vi "L1.1.vi"() -> ()   [LabVIEW 2020]
panel:
  out "Tono 6":dbl
  out "Tono 5":dbl
  out "Tono 4":dbl
  out "Tono 3":dbl
  out "Tono 2":dbl
  out "Tono 1":dbl
  out "DFT (N=64)":dbl[](graph)
  out "6":bool
  out "5":bool
  out "4":bool
  out "3":bool
  out "2":bool
  out "1":bool
  out "DFT (N=512)":dbl[](graph)
  in  "DFT  size":i32=-1
  in  "Canal DA myDAQ":tag="myDAQ1/audioOutputLeft"
  out "error out":errorcluster
  out "myDAQ lectura wav":dbl[](graph)
  in  "Canal AD myDAQ":tag="myDAQ1/audioInputLeft"
  in  "stop":bool
  in  "fs AD (Hz) myDAQ":dbl=50000.0 min=0.0 max=50000.0
  in  "numero de muestras myDAQ":i32
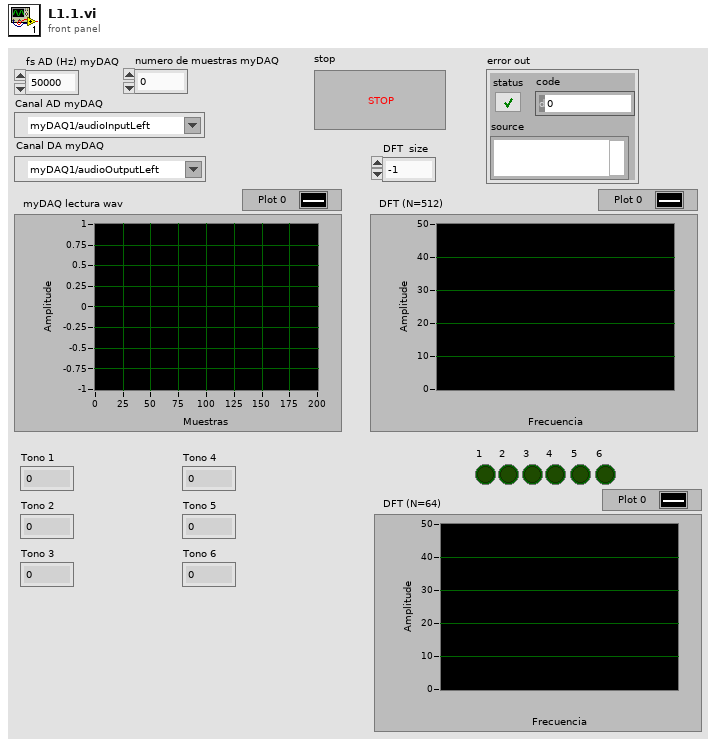
[diagram p1: front panel]
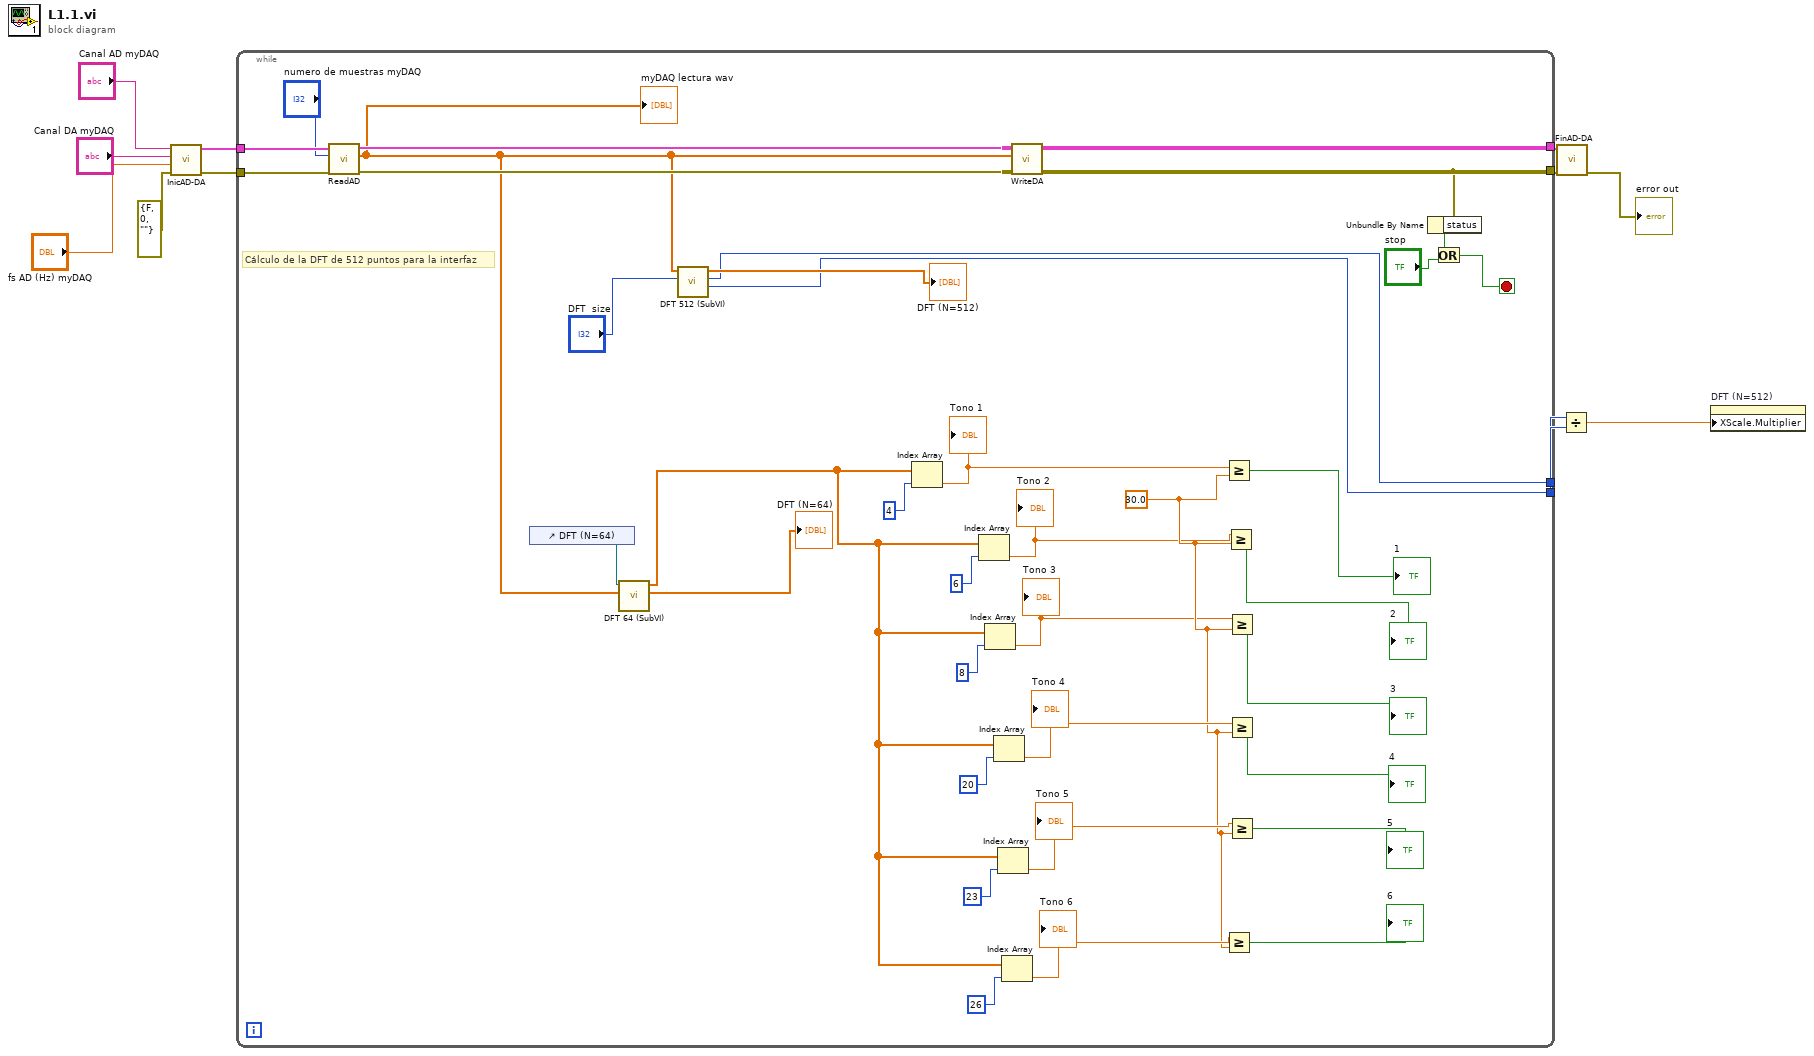
[diagram p0: block diagram]
diagram:
  n1 = call <userlib>:"InicAD-DA.vi"("error in"=errorcluster {"status"=FALSE, "code"=0, "source"=""}, "fs AD (Hz)"="fs AD (Hz) myDAQ", "Canal DA"="Canal DA myDAQ", "Canal AD"="Canal AD myDAQ") -> ("error out"=w9:errorcluster, "Tarea Out"=w10:cluster{"AD":refnum<k21>, "DA":refnum<k21>})  [unwired: 6 in]
  n2 = while {
    tunnel: [w41] -> w12
    tunnel: [w47] -> w11
    tunnel: w10 -> [w46]
    tunnel: w9 -> [w45]
    tunnel: [w38] -> w2
    tunnel: [w37] -> w1
    stop <- w43 stop-if-true
    w24 = 30.0 ("y")
    # "Cálculo de la DFT de 512 puntos para la interfaz"
    n3 = call <userlib>:"ReadAD.vi"("error in"=w45, "numero de muestras"="numero de muestras myDAQ", "Tarea In"=w46) -> ("error out"=w48:errorcluster, "Datos"=w36:dbl[], "Tarea Out"=w49:cluster{"AD":refnum<k21>, "DA":refnum<k21>})  [unwired: 6 in]
    "myDAQ lectura wav" <- w36
    n4 = control-ref of="DFT (N=64)"() -> (w14:refnum<vi>)
    n5 = call "DFT 64 (SubVI).vi"("Datos"=w36, "WaveformGraph in"=w14) -> ("DFT (N=64)"=→"DFT (N=64)":dbl[], "Array"=w29:dbl[])  [unwired: 8 in]
    n6 = call "DFT 512 (SubVI).vi"("DFT  size in"="DFT  size", "Datos"=w36) -> ("DFT  size out"=w38:i32, "x"=w37:i32, "Array"=→"DFT (N=512)":dbl[])  [unwired: 7 in]
    n7 = Index Array(array=w29, index=4) -> (element=w28:dbl)
    "Tono 1" <- w28
    n8 = Index Array(array=w29, index=6) -> (element=w17:dbl)
    "Tono 2" <- w17
    n9 = Index Array(array=w29, index=8) -> (element=w16:dbl)
    "Tono 3" <- w16
    n10 = Index Array(array=w29, index=20) -> (element=w25:dbl)
    "Tono 4" <- w25
    n11 = Index Array(array=w29, index=23) -> (element=w26:dbl)
    "Tono 5" <- w26
    n12 = Index Array(array=w29, index=26) -> (element=w27:dbl)
    "Tono 6" <- w27
    n13 = call <userlib>:"WriteDA.vi"("error in"=w48, "Datos"=w36, "Tarea In"=w49) -> ("error out"=w41:errorcluster, "Tarea Out"=w47:cluster{"AD":refnum<k21>, "DA":refnum<k21>})  [unwired: 7 in]
    n14 = Greater Or Equal?(x=w28, y=w24) -> (x >= y?=→"1":bool)
    n15 = Greater Or Equal?(x=w27, y=w24) -> (x >= y?=→"6":bool)
    n16 = Greater Or Equal?(x=w17, y=w24) -> (x >= y?=→"2":bool)
    n17 = Greater Or Equal?(x=w16, y=w24) -> (x >= y?=→"3":bool)
    n18 = Greater Or Equal?(x=w25, y=w24) -> (x >= y?=→"4":bool)
    n19 = Greater Or Equal?(x=w26, y=w24) -> (x >= y?=→"5":bool)
    n20 = Unbundle By Name(w41) -> ("status"=w40:bool)
    n21 = Or(x=w40, y="stop") -> (x .or. y?=w43:bool)
  }
  n22 = call <userlib>:"FinAD-DA.vi"("error in"=w12, "Tarea In"=w11) -> ("error out"=→"error out":errorcluster)  [unwired: 9 in]
  n23 = Divide(x=w1, y=w2) -> (x/y=w3:dbl)
  n24 = property on="DFT (N=512)" class="WFGraph (strict)"("XScale.Multiplier"=w3) -> ()  [unwired: 2 in, 2 out]
